vi "controls_booleans.vi"(10 "Desired Position":dbl[](array[numeric]) format="%#_13g") -> ()   [LabVIEW 2020]
uses:
  C:/Users/359167/Documents/LabVIEW_ws/Thorlabs.MotionControl.FTD2xx_Net.dll
  Thorlabs.MotionControl.FTD2xx_Net.dll
  <vilib>/Utility/file.llb/Read Delimited Spreadsheet (DBL).vi
  <vilib>/Utility/file.llb/Write Delimited Spreadsheet (DBL).vi
panel:
  in  "Home":bool
  in  "Run":bool
  in  "End":bool
  out "Channel and AP":dbl[][](array[numeric])
  in  "Path 3":path=path "C:/Users/359167/Documents/saved_position.csv"
  in  "Path 2":path=path "C:/Users/359167/Documents/saved_position.csv"
  in  "Path":path=path "C:/Users/359167/Documents/saved_position.csv"
  out "Device ID":string[](array[string])
  out "Serial #":string[](array[string])
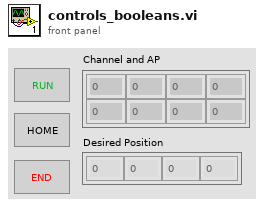
[diagram p1: front panel]
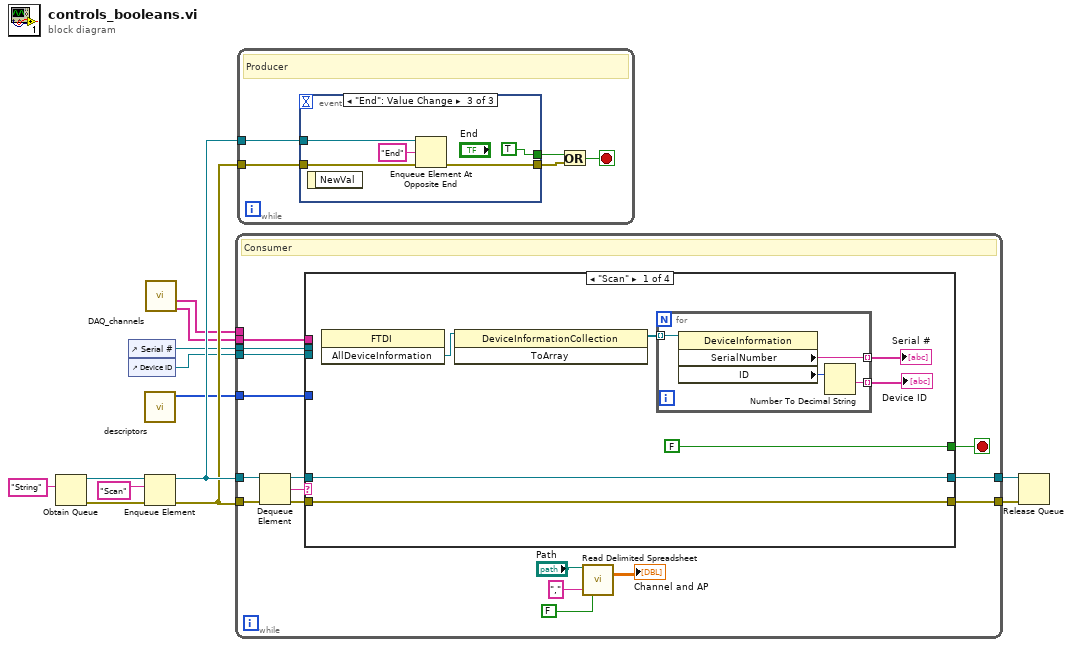
[diagram p0: block diagram]
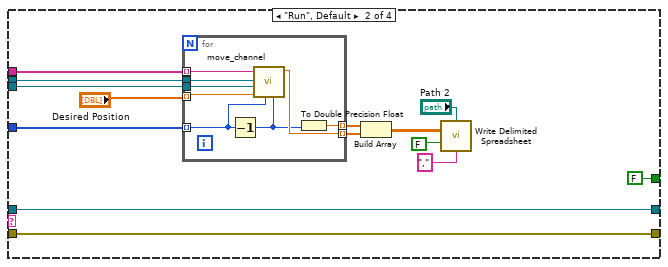
[diagram p2: hidden frame]
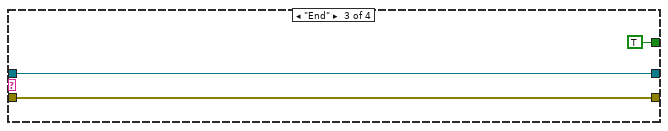
[diagram p3: hidden frame]
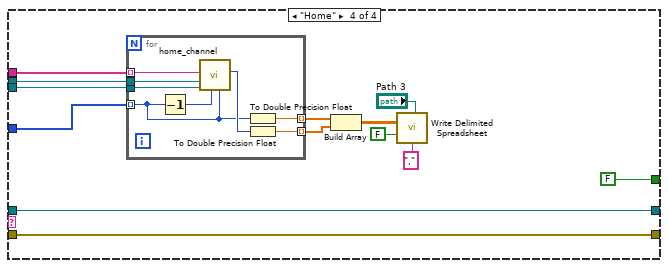
[diagram p4: hidden frame]
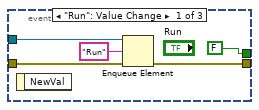
[diagram p5: hidden frame]
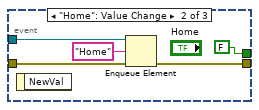
[diagram p6: hidden frame]
diagram:
  n1 = Obtain Queue(element data type="String") -> (queue out=w12:refnum<queue>, error out=w13:errorcluster)  [unwired: 4 in, 1 out]
  n2 = control-ref of="Serial #"() -> (w4:refnum<vi>)
  n3 = control-ref of="Device ID"() -> (w3:refnum<vi>)
  n4 = call "descriptors.vi"() -> ("channel #s"=w5:i32[])  [unwired: 7 in, 4 out]
  n5 = Enqueue Element(queue=w12, element="Scan", error in (no error)=w13) -> (queue out=w10:refnum<queue>, error out=w6:errorcluster)  [unwired: 1 in, 1 out]
  n6 = call "DAQ_channels.vi"() -> ("subset of DAQ channels"=w1:tag[], "all DAQ channels"=w2:tag[])  [unwired: 10 in]
  n7 = while {
    tunnel: w6 -> [w28]
    tunnel: w10 -> [w26]
    tunnel: [w24] -> w7
    tunnel: [w23] -> w8
    tunnel: w1 -> [w18]
    tunnel: w2 -> [_]
    tunnel: w5 -> [w17]
    tunnel: w4 -> [w16]
    tunnel: w3 -> [w15]
    stop <- w14 stop-if-true
    # "Consumer"
    n8 = Dequeue Element(queue=w26, error in (no error)=w28) -> (queue out=w27:refnum<queue>, element=w25:string, error out=w29:errorcluster)  [unwired: 1 in, 1 out]
    n9 = case shown="\"Scan\"" w25 {
      tunnel: [FALSE FALSE TRUE FALSE] -> w14
      tunnel: w29 -> [w30 w54 w63 w77]
      tunnel: w27 -> [w31 w53 w64 w78]
      tunnel: [w30 w54 w63 w77] -> w24
      tunnel: [w31 w53 w64 w78] -> w23
      tunnel: w18 -> [_ w52 _ w76]
      tunnel: w17 -> [_ w44 _ w68]
      tunnel: w16 -> [_ w43 _ w66]
      tunnel: w15 -> [_ w42 _ w67]
      frame "Scan" {
        n10 = invoke class="FTDI" method="AllDeviceInformation"() -> ("AllDeviceInformation"=w36:refnum<k24>)  [unwired: 3 in, 2 out]
        n11 = invoke class="DeviceInformationCollection" method="ToArray"(reference=w36) -> ("ToArray"=w34:refnum<k24>[])  [unwired: 2 in, 2 out]
        n12 = for {
          tunnel: w34 -> [w40] mode=indexing
          tunnel: [w39] -> w32 mode=indexing
          tunnel: [w37] -> w33 mode=indexing
          n13 = property class="DeviceInformation"(reference=w40) -> ("SerialNumber"=w39:string, "ID"=w38:u32)  [unwired: 1 in, 2 out]
          n14 = Number To Decimal String(number=w38) -> (decimal integer string=w37:string)  [unwired: 1 in]
        }
        "Serial #" <- w32
        "Device ID" <- w33
      }
      frame "Run", Default {
        n15 = for {
          tunnel: w52 -> [w58] mode=indexing
          tunnel: "Desired Position" -> [w57] mode=indexing
          tunnel: [w62] -> w47 mode=indexing
          tunnel: [w61] -> w46 mode=indexing
          tunnel: w44 -> [w55] mode=indexing
          tunnel: w43 -> [w59]
          tunnel: w42 -> [w60]
          n16 = Decrement(x=w55) -> (x-1=w56:i32)
          n17 = call "move_channel.vi"("file index"=w56, "Mount Channel"=w55, "Desired"=w57, "Device ID"=w60, "Serial #"=w59, "DAQ Channel"=w58) -> ("Absolute Position"=w62:dbl)  [unwired: 3 in, 2 out]
          n18 = To Double Precision Float(number=w56) -> (double precision float=w61:dbl)
        }
        n19 = Build Array(w46, w47) -> (w45:dbl[][])
        n20 = call-poly <vilib>:"Write Delimited Spreadsheet.vi"("file path (dialog if empty)"="Path 2", "2D data"=w45, "append to file? (new file:F)"=FALSE, "delimiter (\\t)"="," ("delimiter (\\t)")) -> ()  [unwired: 10 in, 2 out]
      }
      frame "End" {
      }
      frame "Home" {
        n21 = for {
          tunnel: w76 -> [w86] mode=indexing
          tunnel: [w85] -> w70 mode=indexing
          tunnel: [w83] -> w69 mode=indexing
          tunnel: w68 -> [w81] mode=indexing
          tunnel: w67 -> [w80]
          tunnel: w66 -> [w79]
          n22 = Decrement(x=w81) -> (x-1=w82:i32)
          n23 = call "home_channel.vi"("Channel"=w81, 6:"DAQ channel"=w82, "Device ID"=w80, "Serial #"=w79, 10:"DAQ channel"=w86) -> ("Zero"=w84:i32)  [unwired: 5 in, 1 out]
          n24 = To Double Precision Float(number=w81) -> (double precision float=w85:dbl)
          n25 = To Double Precision Float(number=w84) -> (double precision float=w83:dbl)
        }
        n26 = Build Array(w70, w69) -> (w72:dbl[][])
        n27 = call-poly <vilib>:"Write Delimited Spreadsheet.vi"("file path (dialog if empty)"="Path 3", "2D data"=w72, "append to file? (new file:F)"=FALSE, "delimiter (\\t)"="," ("delimiter (\\t)")) -> ()  [unwired: 10 in, 2 out]
      }
    }
    n28 = call-poly <vilib>:"Read Delimited Spreadsheet.vi"("file path (dialog if empty)"="Path", "transpose? (F)"=FALSE, "delimiter (\\t)"="," ("delimiter (\\t)")) -> ("all rows"=→"Channel and AP":dbl[][])  [unwired: 7 in, 5 out]
  }
  n29 = while {
    tunnel: w10 -> [w90]
    tunnel: w6 -> [w89]
    stop <- w91 stop-if-true
    # "Producer"
    n30 = event shown="[2] \"End\": Value Change" {
      selector: _ -> [_ _ _]
      dyn-events: _ -> [_ _ _]
      timeout: _ -> [_ _ _]
      tunnel: [FALSE ("End") FALSE ("End") TRUE ("End")] -> w88
      tunnel: w90 -> [w96 w100 w106]
      tunnel: w89 -> [w94 w99 w104]
      tunnel: [w92 w97 w102] -> w87
      event "Run": Value Change {
        n31 = event-data() -> ()  [unwired: 1 in, 1 out]
        n32 = Enqueue Element(queue=w96, element="Run", error in (no error)=w94) -> (error out=w92:errorcluster)  [unwired: 1 in, 2 out]
      }
      event "Home": Value Change {
        n33 = event-data() -> ()  [unwired: 1 in, 1 out]
        n34 = Enqueue Element(queue=w100, element="Home", error in (no error)=w99) -> (error out=w97:errorcluster)  [unwired: 1 in, 2 out]
      }
      event "End": Value Change {
        n35 = event-data() -> ()  [unwired: 1 in, 1 out]
        n36 = Enqueue Element At Opposite End(queue=w106, element="End", error in (no error)=w104) -> (error out=w102:errorcluster)  [unwired: 1 in, 2 out]
      }
    }
    n37 = Or(x=w88, y=w87) -> (x .or. y?=w91:bool)
  }
  n38 = Release Queue(queue=w8, error in (no error)=w7) -> ()  [unwired: 1 in, 3 out]
